vi "Initial_Menu.vi"() -> ()   [LabVIEW 2020]
panel:
  in  "Guide Button":bool
  in  "End Button":bool
  in  "Sinc Mode":bool
  in  "Master Mode":bool
  # "DPO70000SX Series Oscilloscopes- Tektronix"
  # "CHOOSE THE OSCILLOSCOPES MODE THAT YOU PREFER"
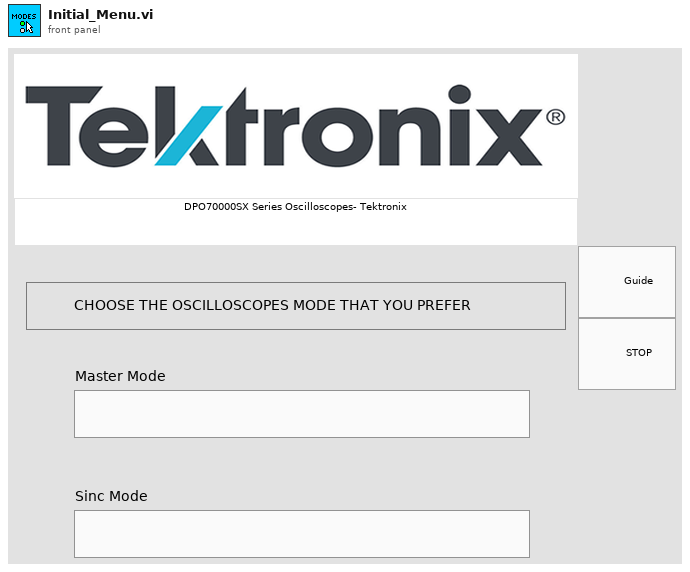
[diagram p1: front panel]
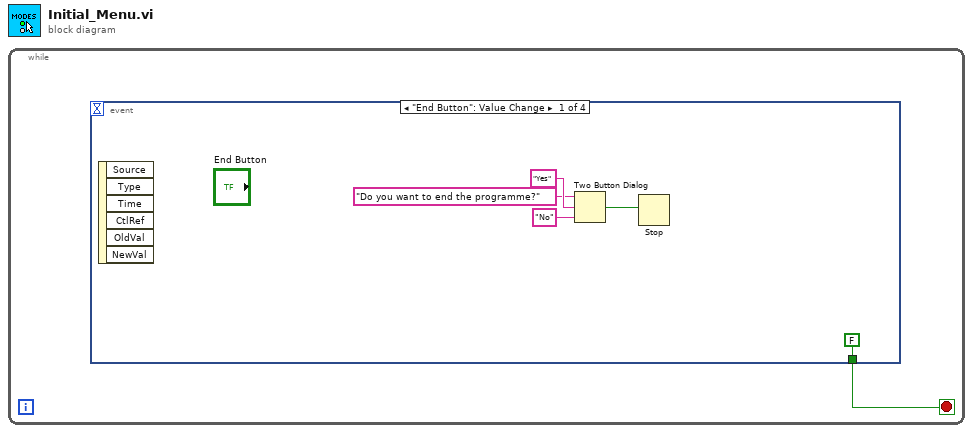
[diagram p0: block diagram]
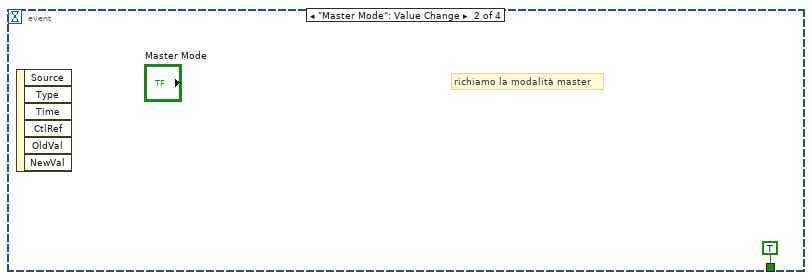
[diagram p2: hidden frame]
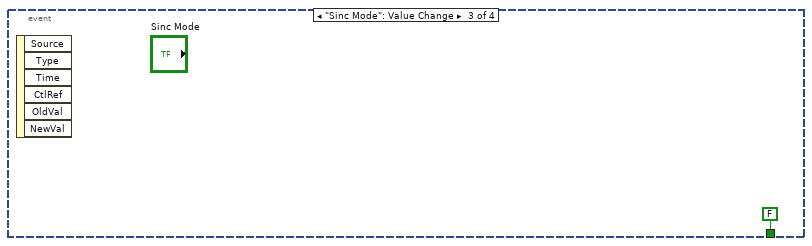
[diagram p3: hidden frame]
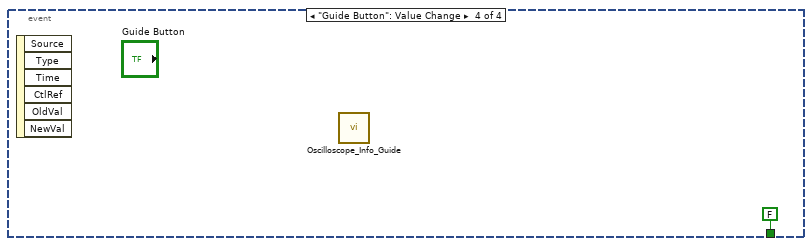
[diagram p4: hidden frame]
diagram:
  n1 = while {
    stop <- w1 stop-if-true
    n2 = event shown="[0] \"End Button\": Value Change" {
      selector: _ -> [_ _ _ _]
      dyn-events: _ -> [_ _ _ _]
      timeout: _ -> [_ _ _ _]
      tunnel: [FALSE TRUE FALSE FALSE] -> w1
      event "End Button": Value Change {
        n3 = event-data() -> ()  [unwired: 1 in, 6 out]
        n4 = Two Button Dialog(message="Do you want to end the programme?", 1:"No" ("F button name (\"Cancel\")"), 2:"Yes" ("T button name (\"OK\")")) -> (T button?=w2:bool)
        n5 = Stop(stop? (T)=w2) -> ()
      }
      event "Master Mode": Value Change {
        # "richiamo la modalità master"
        n6 = event-data() -> ()  [unwired: 1 in, 6 out]
      }
      event "Sinc Mode": Value Change {
        n7 = event-data() -> ()  [unwired: 1 in, 6 out]
      }
      event "Guide Button": Value Change {
        n8 = event-data() -> ()  [unwired: 1 in, 6 out]
        n9 = call "Oscilloscope_Info_Guide.vi"() -> ()  [unwired: 12 in]
      }
    }
  }
